vi "Feeder.vi"(11 "SHOOT Button":bool) -> (3 "Ready To Shoot?":bool)   [LabVIEW 2012]
uses:
  <vilib>/Rock Robotics/WPI/Solenoid/Deprecated/WPI_SolenoidSetBool.vi
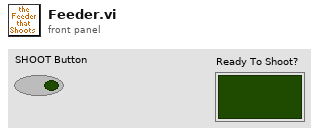
[diagram p1: front panel]
types:
  T1 = typedef "WPI_SolenoidDevRef.ctl" = cluster{"DevStatus":errorcluster, "Solenoid Module":T2, "Forward Solenoid Channel":T3, "Reverse Solenoid Channel":T3}
  T2 = typedef "FPGA_TypedefSolenoidModule.ctl" = enum16{"Solenoid Module 1", "Solenoid Module 2"}
  T3 = typedef "WPI_SolenoidChannel.ctl" = enum8{"Solenoid 1", "Solenoid 2", "Solenoid 3", "Solenoid 4", "Solenoid 5", "Solenoid 6", "Solenoid 7", "Solenoid 8", "Invalid"}
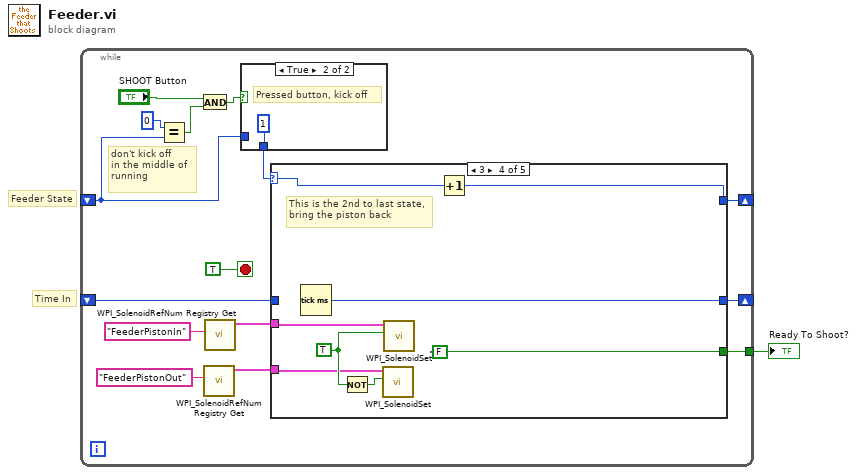
[diagram p0: block diagram]
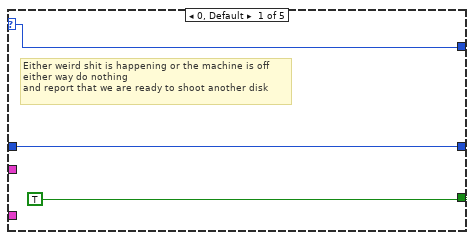
[diagram p2: hidden frame]
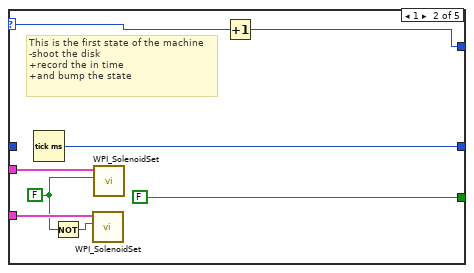
[diagram p3: hidden frame]
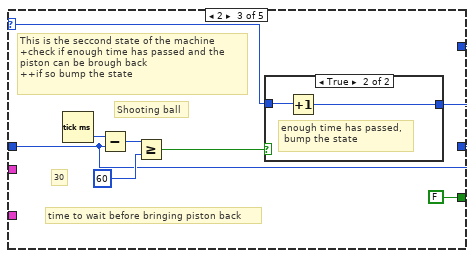
[diagram p4: hidden frame]
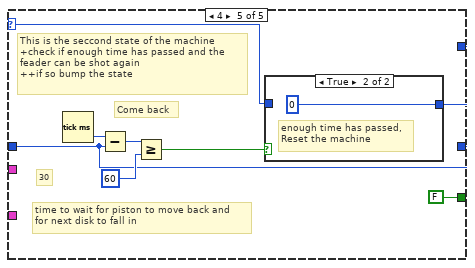
[diagram p6: hidden frame]
diagram:
  # "Feeder State"
  # "Time In"
  n1 = while {
    tunnel: [w14] -> w1
    shift-right: [w8] -> _
    shift-left: _ -> [w10]
    shift-right: [w9] -> _
    shift-left: _ -> [w3]
    stop <- TRUE stop-if-true
    # "don't kick off\nin the middle of\nrunning"
    n2 = Equal?(x=0, y=w3) -> (x = y?=w5:bool)
    n3 = And(x="SHOOT Button", y=w5) -> (x .and. y?=w4:bool)
    n4 = call <vilib>:"WPI_SolenoidRefNum Registry Get.vi"("refnum name"="FeederPistonOut") -> ("SolenoidDevRef"=w12:T1)  [unwired: 9 in, 1 out]
    n5 = call <vilib>:"WPI_SolenoidRefNum Registry Get.vi"("refnum name"="FeederPistonIn") -> ("SolenoidDevRef"=w13:T1)  [unwired: 9 in, 1 out]
    n6 = case shown="True" w4 {
      tunnel: [w57 1] -> w2
      tunnel: w3 -> [w57 _]
      frame False {
        # "Not pressed button"
      }
      frame True {
        # "Pressed button, kick off"
      }
    }
    n7 = case shown="3" w2 {
      selector: w2 -> [w17 w20 w28 w39 w47]
      tunnel: [TRUE FALSE FALSE FALSE FALSE] -> w14
      tunnel: w13 -> [_ w26 _ w44 _]
      tunnel: w12 -> [_ w25 _ w43 _]
      tunnel: w10 -> [w18 _ w29 _ w48]
      tunnel: [w17 w21 w30 w40 w49] -> w9
      tunnel: [w18 w22 w29 w41 w48] -> w8
      frame 0, Default {
        # "Either weird shit is happening or the machine is off\neither way do nothing\nand report that we are ready to shoot another disk"
      }
      frame 1 {
        w23 = FALSE
        # "This is the first state of the machine\n-shoot the disk\n+record the in time\n+and bump the state"
        n8 = Tick Count (ms)() -> (millisecond timer value=w22:u32)
        n9 = Not(x=w23) -> (.not. x?=w24:bool)
        n10 = call-poly <vilib>:"WPI_SolenoidSet.vi"("Value"=w24, "SolenoidDevRef"=w25) -> ()  [unwired: 8 in, 2 out]
        n11 = call-poly <vilib>:"WPI_SolenoidSet.vi"("Value"=w23, "SolenoidDevRef"=w26) -> ()  [unwired: 8 in, 2 out]
        n12 = Increment(x=w20) -> (x+1=w21:i32)
      }
      frame 2 {
        # "time to wait before bringing piston back"
        # "30"
        # "Shooting ball"
        # "This is the seccond state of the machine\n+check if enough time has passed and the \npiston can be brough back\n++if so bump the state"
        n13 = Tick Count (ms)() -> (millisecond timer value=w35:u32)
        n14 = Subtract(x=w35, y=w29) -> (x-y=w34:u32)
        n15 = Greater Or Equal?(x=w34, y=60 ("Ms to wait piston in")) -> (x >= y?=w31:bool)
        n16 = case shown="True" w31 {
          tunnel: w28 -> [w36 w37]
          tunnel: [w36 w38] -> w30
          frame False {
            # "not enough time has passed,\n don't do anything"
          }
          frame True {
            # "enough time has passed,\n bump the state"
            n17 = Increment(x=w37) -> (x+1=w38:i32)
          }
        }
      }
      frame 3 {
        w45 = TRUE
        # "This is the 2nd to last state,\nbring the piston back"
        n18 = Tick Count (ms)() -> (millisecond timer value=w41:u32)
        n19 = Not(x=w45) -> (.not. x?=w46:bool)
        n20 = call-poly <vilib>:"WPI_SolenoidSet.vi"("Value"=w46, "SolenoidDevRef"=w43) -> ()  [unwired: 8 in, 2 out]
        n21 = call-poly <vilib>:"WPI_SolenoidSet.vi"("Value"=w45, "SolenoidDevRef"=w44) -> ()  [unwired: 8 in, 2 out]
        n22 = Increment(x=w39) -> (x+1=w40:i32)
      }
      frame 4 {
        # "time to wait for piston to move back and\nfor next disk to fall in"
        # "30"
        # "Come back"
        # "This is the seccond state of the machine\n+check if enough time has passed and the \nfeader can be shot again\n++if so bump the state"
        n23 = Tick Count (ms)() -> (millisecond timer value=w54:u32)
        n24 = Subtract(x=w54, y=w48) -> (x-y=w53:u32)
        n25 = Greater Or Equal?(x=w53, y=60 ("Ms to wait piston out (disk down)")) -> (x >= y?=w50:bool)
        n26 = case shown="True" w50 {
          tunnel: w47 -> [w55 _]
          tunnel: [w55 0] -> w49
          frame False {
            # "not enough time has passed,\n don't do anything"
          }
          frame True {
            # "enough time has passed,\nReset the machine"
          }
        }
      }
    }
  }
  "Ready To Shoot?" <- w1
